vi "Dialog Box - Two Button.vi"(4 "False Button Text (Cancel)":string="Cancel", 5 "Key Focus":enum16{"None", "True", "False"}(ring), 6 "True Button Text (Continue)":string="Continue", 7 "Timeout (Seconds)":i16=-1, 8 "error in (no error)":errorcluster, 11 "Text":string) -> (0 "error out":errorcluster, 1 "Timeout":bool, 2 "False Button":bool, 3 "True Button":bool)   [LabVIEW 2011]
doc: "Displays a simple two button dialog box.\n\nA timeout can be set. If no timeout is defined then the dialog will wait forever.\nThe text for each button can be set.\nEither button can receive key focus."
panel:
  in  "FALSE Button":bool
  in  "TRUE Button":bool
  out "String":string
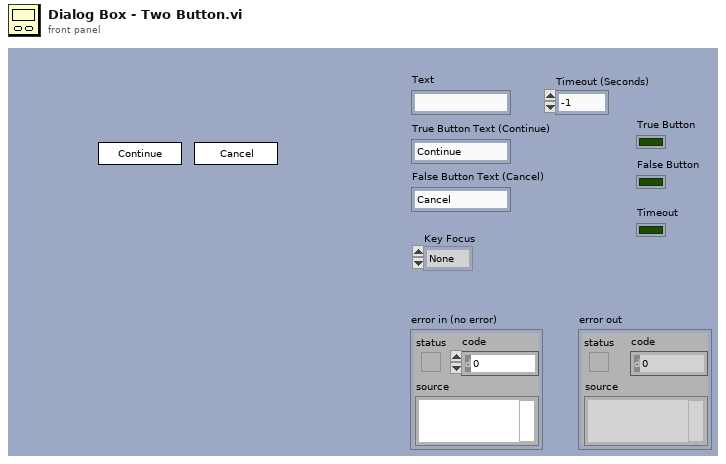
[diagram p1: front panel]
types:
  T1 = enum32{"Invalid", "Default", "Floating", "Floating/Auto-Hide", "Modal"}
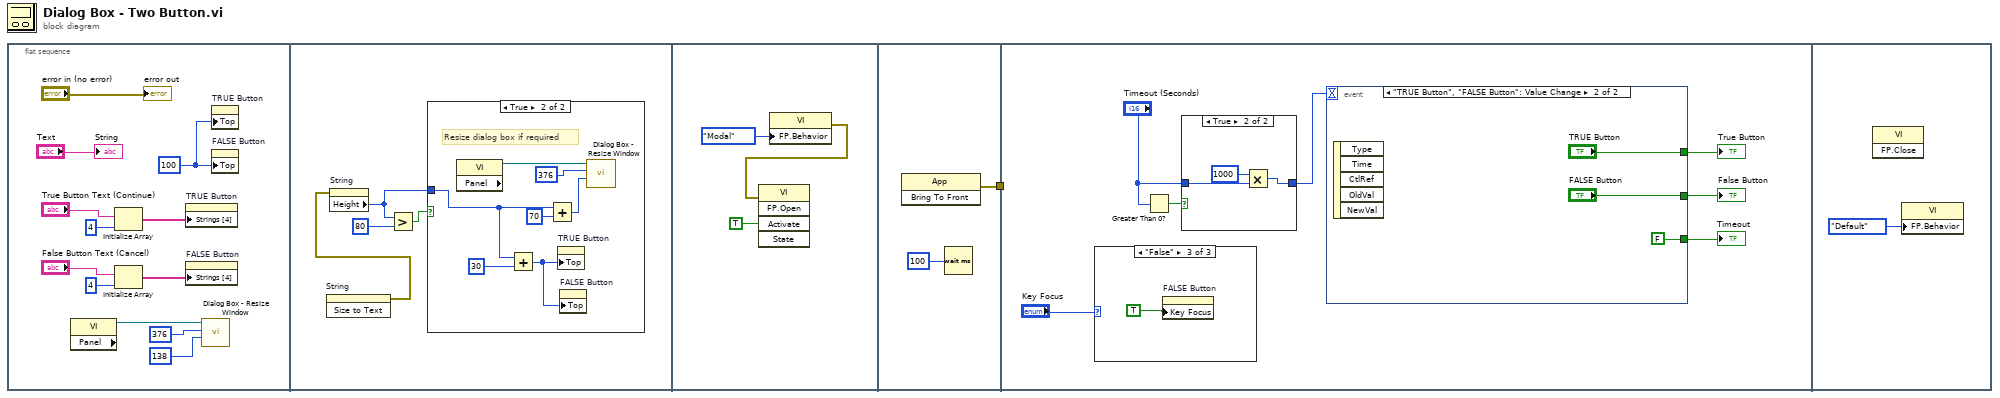
[diagram p0: block diagram]
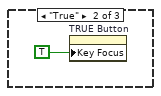
[diagram p4: hidden frame]
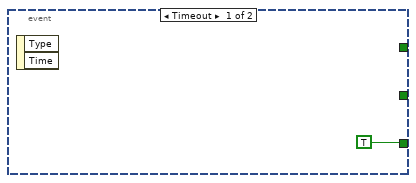
[diagram p5: hidden frame]
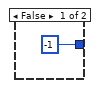
[diagram p6: hidden frame]
diagram:
  n1 = flat-sequence {
    tunnel: [w29] -> w1
    tunnel: w1 -> [_]
    frame #0 {
      w2 = 100 ("Position:Top")
      n2 = property class="VI" props=["Panel"]() -> (reference out=w5:refnum<vi>)  [unwired: 2 in, 2 out]
      n3 = Initialize Array("True Button Text (Continue)", 4 ("dimension size")) -> (w6:string[])
      n4 = Initialize Array("False Button Text (Cancel)", 4 ("dimension size")) -> (w7:string[])
      n5 = property on="TRUE Button" class="Bool"("Strings [4]"=w6) -> ()  [unwired: 2 in, 2 out]
      n6 = property on="FALSE Button" class="Bool"("Strings [4]"=w7) -> ()  [unwired: 2 in, 2 out]
      n7 = call "Dialog Box - Resize Window.vi"("Height"=i16 138, "Width"=i16 376, "reference"=w5) -> ()  [unwired: 8 in, 1 out]
      n8 = property on="TRUE Button" class="Bool"("Top"=w2) -> ()  [unwired: 2 in, 2 out]
      n9 = property on="FALSE Button" class="Bool"("Top"=w2) -> ()  [unwired: 2 in, 2 out]
      "String" <- "Text"
      "error out" <- "error in (no error)"
    }
    frame #1 {
      n10 = invoke on="String" class="Str" method="Size to Text"() -> (error out=w17:errorcluster)  [unwired: 3 in, 2 out]
      n11 = property on="String" class="Str"(error in=w17) -> ("Height"=w16:u32)  [unwired: 1 in, 2 out]
      n12 = Greater?(x=w16, y=u32 80) -> (0:w15:bool)
      n13 = case shown="True" w15 {
        tunnel: w16 -> [_ w20]
        frame False {
        }
        frame True {
          # "Resize dialog box if required"
          n14 = property class="VI" props=["Panel"]() -> (reference out=w24:refnum<vi>)  [unwired: 2 in, 2 out]
          n15 = Add(x=w20, y=u32 30) -> (x+y=w18:u32)
          n16 = Add(x=w20, y=u32 70) -> (x+y=w22:u32)
          n17 = property on="TRUE Button" class="Bool"("Top"=w18) -> ()  [unwired: 2 in, 2 out]
          n18 = property on="FALSE Button" class="Bool"("Top"=w18) -> ()  [unwired: 2 in, 2 out]
          n19 = call "Dialog Box - Resize Window.vi"("Height"=w22, "Width"=i16 376, "reference"=w24) -> ()  [unwired: 8 in, 1 out]
        }
      }
    }
    frame #2 {
      n20 = property class="VI"("FP.Behavior"=T1."Modal" ("Front Panel Window:Behavior")) -> (error out=w25:errorcluster)  [unwired: 2 in, 1 out]
      n21 = invoke class="VI" method="FP.Open"(error in=w25, "Activate"=TRUE ("Activate?")) -> ()  [unwired: 3 in, 5 out]
    }
    frame #3 {
      n22 = invoke class="App" method="Bring To Front"() -> (error out=w29:errorcluster)  [unwired: 3 in, 2 out]
      n23 = Wait (ms)(milliseconds to wait=u32 100) -> ()  [unwired: 1 out]
    }
    frame #4 {
      n24 = case shown="\"False\"" "Key Focus" {
        frame "None", Default {
        }
        frame "True" {
          n25 = property on="TRUE Button" class="Bool"("Key Focus"=TRUE) -> ()  [unwired: 2 in, 2 out]
        }
        frame "False" {
          n26 = property on="FALSE Button" class="Bool"("Key Focus"=TRUE) -> ()  [unwired: 2 in, 2 out]
        }
      }
      n27 = Greater Than 0?(x="Timeout (Seconds)") -> (x > 0?=w35:bool)
      n28 = case shown="True" w35 {
        tunnel: "Timeout (Seconds)" -> [_ w44]
        tunnel: [i16 -1 w45] -> w34
        frame False {
        }
        frame True {
          n29 = Multiply(x=i16 1000, y=w44) -> (x*y=w45:i16)
        }
      }
      n30 = event shown="[1] \"TRUE Button\", \"FALSE Button\": Value Change" {
        selector: _ -> [_ _]
        dyn-events: _ -> [_ _]
        timeout: w34 -> [_ _]
        tunnel: [_ "TRUE Button"] -> w33
        tunnel: [_ "FALSE Button"] -> w32
        tunnel: [TRUE FALSE] -> w31
        event Timeout {
          n31 = event-data() -> ()  [unwired: 1 in, 2 out]
        }
        event "TRUE Button", "FALSE Button": Value Change {
          n32 = event-data() -> ()  [unwired: 1 in, 5 out]
        }
      }
      "True Button" <- w33
      "False Button" <- w32
      "Timeout" <- w31
    }
    frame #5 {
      n33 = invoke class="VI" method="FP.Close"() -> ()  [unwired: 3 in, 3 out]
      n34 = property class="VI"("FP.Behavior"=T1."Default" ("Front Panel Window:Behavior")) -> ()  [unwired: 2 in, 2 out]
    }
  }
